vi "NanotecSMCPDDriver.check internal errors.vi"(0 "VISA resource name":refnum<visa-resource-name>, 1 "contollerID":i32=-1, 5 "error in (no error)":errorcluster) -> (14 "VISA resource name out":refnum<visa-resource-name>, 15 "contollerID out":i32=-1, 16 "Error Code":i32[](array[numeric]), 17 "Error Message":string, 19 "error out":errorcluster)   [LabVIEW 2014, in "NanotecSMCPDDriver.lvlib"]
doc: "Queries the instrument for internal errors. These are typically unrelated to commands sent to the instrument. But may stay in the error registers for a long time. Typically, starting up a controller causes some errors to \"hang around\" for a long time.\n\nAn application should just check from time to time, if the \"error pattern\" has changed."
uses:
  NanotecSMCPDDriver.lvlib
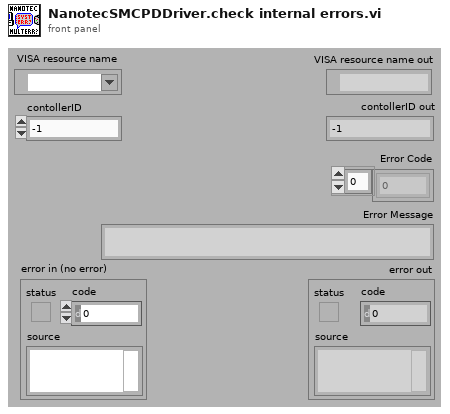
[diagram p1: front panel]
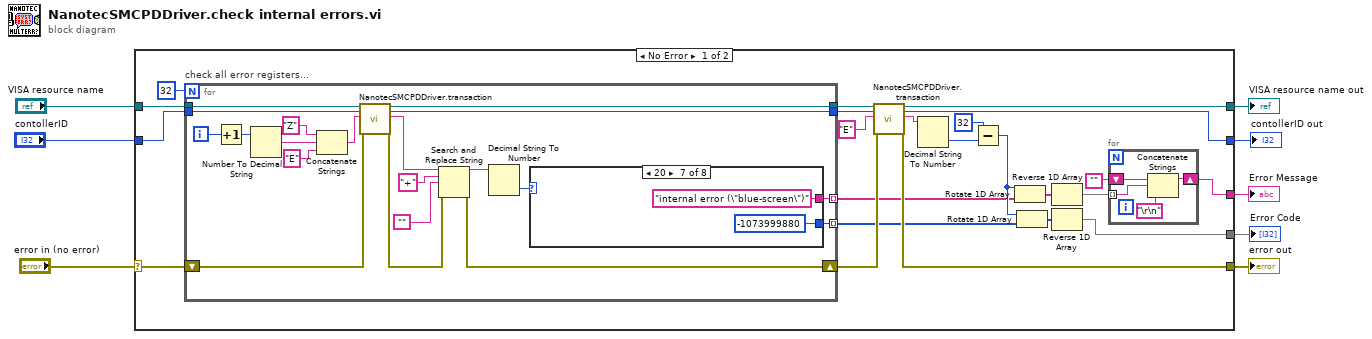
[diagram p0: block diagram]
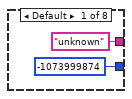
[diagram p2: hidden frame]
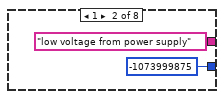
[diagram p3: hidden frame]
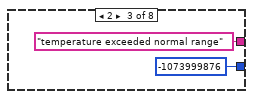
[diagram p4: hidden frame]
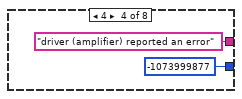
[diagram p5: hidden frame]
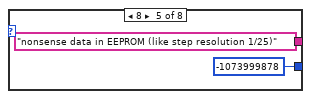
[diagram p6: hidden frame]
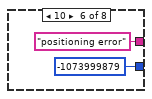
[diagram p7: hidden frame]
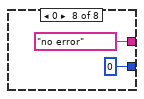
[diagram p8: hidden frame]
diagram:
  n1 = case "error?" shown="No Error" "error in (no error)" {
    selector: "error in (no error)" -> [w29 w72]
    tunnel: [w16 w74] -> w8
    tunnel: "VISA resource name" -> [w31 w74]
    tunnel: [w22 w72] -> w6
    tunnel: "contollerID" -> [w30 w73]
    tunnel: [w17 w73] -> w4
    tunnel: [w9 _] -> w2
    tunnel: [w18 _] -> w1
    frame No Error {
      n2 = for "check all error registers..." {
        N: 32 -> [_]
        tunnel: w31 -> [w55]
        tunnel: [w54] -> w27
        tunnel: w30 -> [w53]
        tunnel: [w52] -> w26
        shift-right: [w36] -> w23
        shift-left: w29 -> [w51]
        tunnel: [w41] -> w11 mode=indexing
        tunnel: [w40] -> w12 mode=indexing
        i -> [w39]
        n3 = Increment(x=w39) -> (x+1=w50:i32)
        n4 = Number To Decimal String(number=w50) -> (decimal integer string=w48:string)  [unwired: 1 in]
        n5 = Concatenate Strings("Z" ("string"), w48, "E" ("string")) -> (w46:string)
        n6 = call "NanotecSMCPDDriver.transaction.vi"("VISAresource"=w55, "contollerID"=w53, "commandString"=w46, "error in (no error)"=w51) -> ("VISAresource out"=w54:refnum<visa-resource-name>, "contollerID out"=w52:i32, "response"=w45:string, "error out"=w37:errorcluster)  [unwired: 10 in, 2 out]
        n7 = Search and Replace String(input string=w45, search string="+", replace string="" ("replace string (\"\")"), error in=w37) -> (result string=w43:string, error out=w36:errorcluster)  [unwired: 4 in, 2 out]
        n8 = Decimal String To Number(string=w43) -> (number=w42:i32)  [unwired: 2 in, 1 out]
        n9 = case shown="20" w42 {
          tunnel: ["unknown" "low voltage from power supply" "temperature exceeded normal range" "driver (amplifier) reported an error" "nonsense data in EEPROM (like step resolution 1/25)" "positioning error" "internal error (\"blue-screen\")" "no error"] -> w40
          tunnel: [-1073999874 -1073999875 -1073999876 -1073999877 -1073999878 -1073999879 -1073999880 0] -> w41
          frame Default {
          }
          frame 1 {
          }
          frame 2 {
          }
          frame 4 {
          }
          frame 8 {
          }
          frame 10 {
          }
          frame 20 {
          }
          frame 0 {
          }
        }
      }
      n10 = call "NanotecSMCPDDriver.transaction.vi"("VISAresource"=w27, "contollerID"=w26, "commandString"="E", "error in (no error)"=w23) -> ("VISAresource out"=w16:refnum<visa-resource-name>, "contollerID out"=w17:i32, "response"=w24:string, "error out"=w22:errorcluster)  [unwired: 10 in, 2 out]
      n11 = Decimal String To Number(string=w24) -> (number=w13:i32)  [unwired: 2 in, 1 out]
      n12 = Subtract(x=32, y=w13) -> (x-y=w15:i32)
      n13 = Rotate 1D Array(1:w12, 2:w15) -> (0:w20:string[])
      n14 = Rotate 1D Array(1:w11, 2:w15) -> (0:w21:i32[])
      n15 = Reverse 1D Array(array=w20) -> (reversed array=w10:string[])
      n16 = Reverse 1D Array(array=w21) -> (reversed array=w9:i32[])
      n17 = for {
        tunnel: w10 -> [w33] mode=indexing
        shift-right: [w34] -> w18
        shift-left: "" ("Empty String Constant") -> [w35]
        n18 = Concatenate Strings(w35, w33, "\r\n" ("End of Line Constant")) -> (w34:string)
      }
    }
    frame Error {
    }
  }
  "VISA resource name out" <- w8
  "error out" <- w6
  "Error Message" <- w1
  "Error Code" <- w2
  "contollerID out" <- w4
